vi "Unit Label Setter.vi"(10 "Input String":string, 11 "Label Type":T1) -> (2 "Output String":string)   [LabVIEW 2013]
uses:
  Apps/Unit Label Type.ctl
  Data Access Objects/Metadata/Persistant DAO Actions.ctl
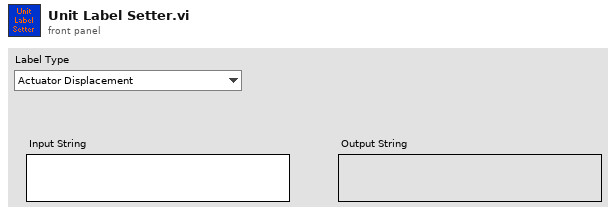
[diagram p1: front panel]
types:
  T1 = typedef "Unit Label Type.ctl" = enum16{"Actuator Displacement", "Actuator Force", "Cartesian Force", "Cartesian Translation", "Cartesian Rotation", "Cartesian Moment"}
  T2 = typedef "Persistant DAO Actions.ctl" = enum16{"Init", "Get", "Set", "Load", "Save"}
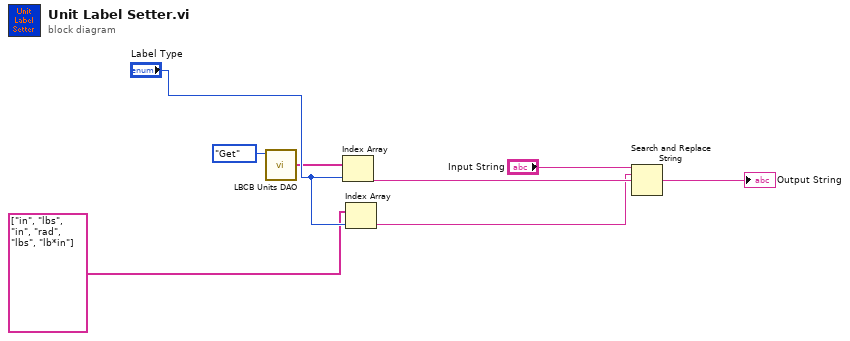
[diagram p0: block diagram]
diagram:
  n1 = call "LBCB Units DAO.vi"("Persistent DAO Actions"=Persistant_DAO_Actions."Get") -> ("Unit Labels Out"=w3:string[])  [unwired: 6 in, 4 out]
  n2 = Index Array(array=w3, index="Label Type") -> (element=w2:string)
  n3 = Index Array(array=string[] ["in", "lbs", "in", "rad", "lbs", "lb*in"], index="Label Type") -> (element=w1:string)
  n4 = Search and Replace String(input string="Input String", search string=w1, replace string=w2) -> (result string=→"Output String":string)  [unwired: 5 in, 3 out]
